vi "Curtin_FixJson.vi"(11 "String In":string) -> (3 "String out":string)   [LabVIEW 2022 SP3]
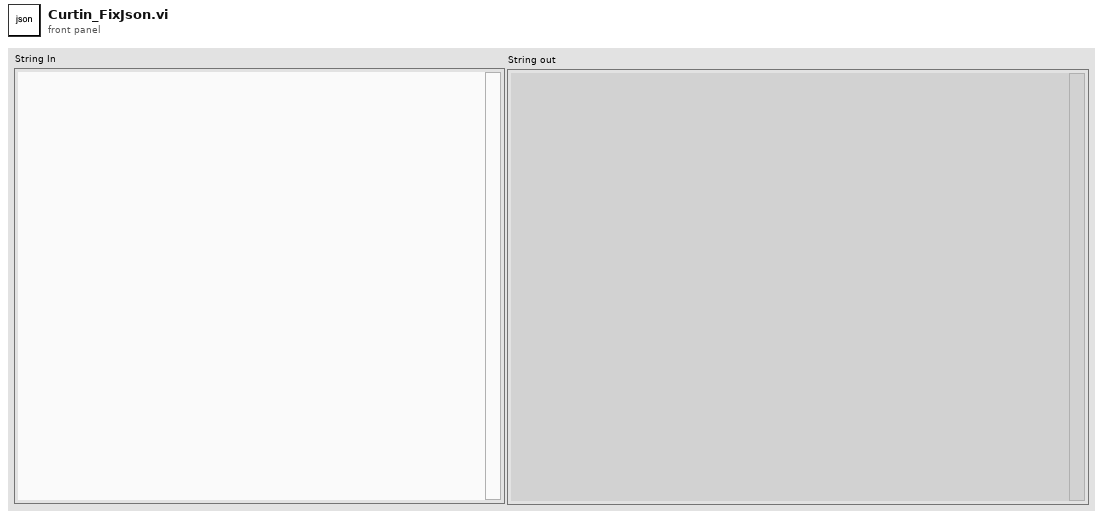
[diagram p1: front panel]
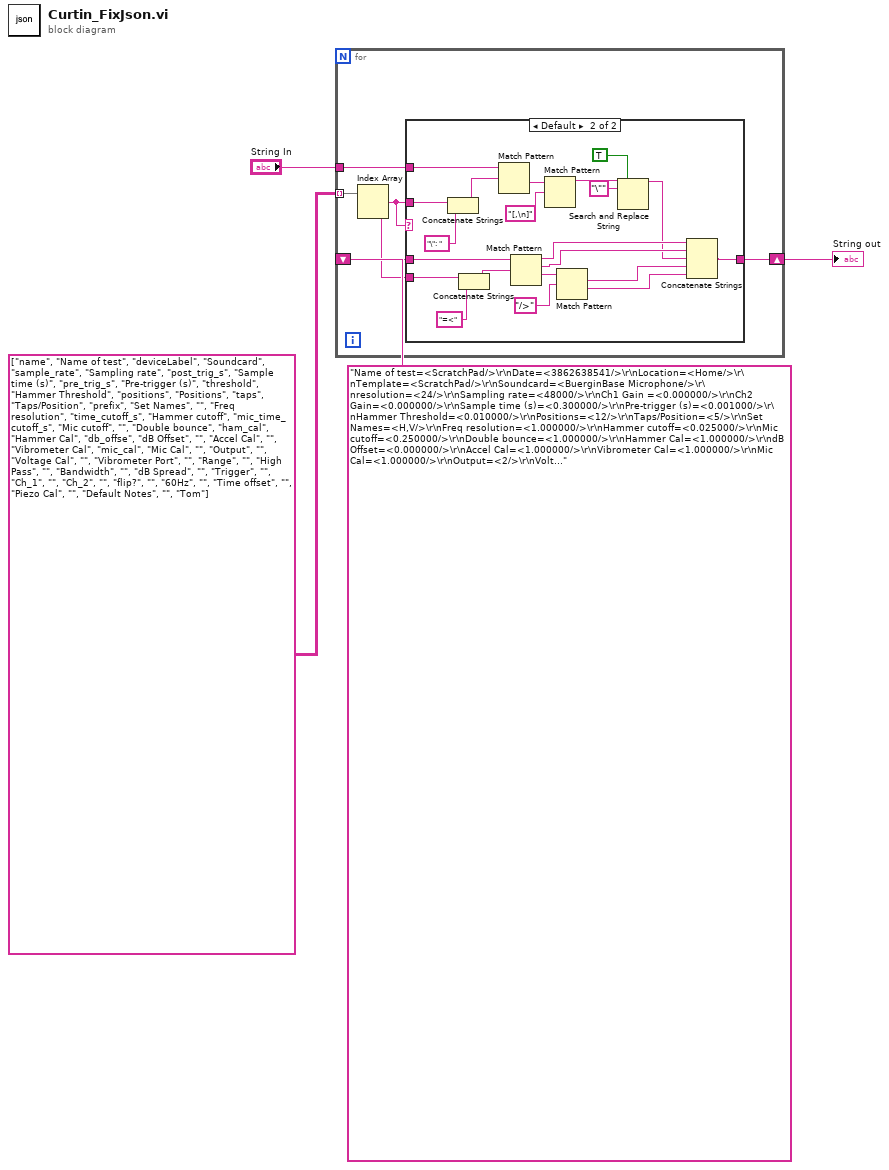
[diagram p0: block diagram]
diagram:
  n1 = for {
    tunnel: "String In" -> [w10]
    tunnel: string[][] [["name", "Name of test"], ["deviceLabel", "Soundcard"], ["sample_rate", "Sampling rate"], ["post_trig_s", "Sample time (s)"], ["pre_trig_s", "Pre-trigger (s)"], ["threshold", "Hammer Threshold"], ["positions", "Positions"], ["taps", "Taps/Position"], ["prefix", "Set Names"], ["", "Freq resolution"], ["time_cutoff_s", "Hammer cutoff"], ["mic_time_cutoff_s", "Mic cutoff"], ["", "Double bounce"], ["ham_cal", "Hammer Cal"], ["db_offse", "dB Offset"], ["", "Accel Cal"], ["", "Vibrometer Cal"], ["mic_cal", "Mic Cal"], ["", "Output"], ["", "Voltage Cal"], ["", "Vibrometer Port"], ["", "Range"], ["", "High Pass"], ["", "Bandwidth"], ["", "dB Spread"], ["", "Trigger"], ["", "Ch_1"], ["", "Ch_2"], ["", "flip?"], ["", "60Hz"], ["", "Time offset"], ["", "Piezo Cal"], ["", "Default Notes"], ["", "Tom"]] -> [w9] mode=indexing
    shift-right: [w6] -> w1
    shift-left: "Name of test=<ScratchPad/>\r\nDate=<3862638541/>\r\nLocation=<Home/>\r\nTemplate=<ScratchPad/>\r\nSoundcard=<BuerginBase Microphone/>\r\nresolution=<24/>\r\nSampling rate=<48000/>\r\nCh1 Gain =<0.000000/>\r\nCh2 Gain=<0.000000/>\r\nSample time (s)=<0.300000/>\r\nPre-trigger (s)=<0.001000/>\r\nHammer Threshold=<0.010000/>\r\nPositions=<12/>\r\nTaps/Position=<5/>\r\nSet Names=<H,V/>\r\nFreq resolution=<1.000000/>\r\nHammer cutoff=<0.025000/>\r\nMic cutoff=<0.250000/>\r\nDouble bounce=<1.000000/>\r\nHammer Cal=<1.000000/>\r\ndB Offset=<0.000000/>\r\nAccel Cal=<1.000000/>\r\nVibrometer Cal=<1.000000/>\r\nMic Cal=<1.000000/>\r\nOutput=<2/>\r\nVoltage Cal=<1.000000/>\r\nVibrometer Port=<ASRL27::INSTR/>\r\nRange=<50/>\r\nHigh Pass=<2/>\r\nBandwidth=<25/>\r\nX Range=<2.000000E+2\t1.000000E+4\t1.000000E+1\t1.000000E+2\t2.000000E+2\n0.000000E+0\t5.000000E-2\t2.500000E-2\t2.500000E-3\t0.000000E+0\n0.000000E+0\t3.000000E-1\t1.000000E-1\t1.000000E-2\t0.000000E+0\n2.000000E+2\t1.000000E+4\t1.000000E+1\t1.000000E+2\t1.000000E+3\n/>\r\nY Range=<-2.500000E+1\t0.000000E+0\t5.000000E+0\t1.000000E+0\t-2.500000E+1\n-1.000000E-1\t1.000000E+0\t2.500000E-1\t5.000000E-2\t0.000000E+0\n-1.000000E+0\t1.000000E+0\t5.000000E-1\t1.000000E-1\t-1.000000E+0\n-1.100000E+1\t2.900000E+1\t2.000000E+0\t5.000000E-1\t-1.000000E+1\n/>\r\ndB Spread=<40.000000/>\r\nTrigger=<0/>\r\nCh_1=<2/>\r\nCh_2=<1/>\r\nflip?=<false/>\r\n60Hz=<false/>\r\nTime offset=<0.000000/>\r\nPiezo Cal=<1.000000/>\r\nDefault Notes=<Instrument info: \n\n\n \nTemplate: HV 24  Obie 26\n\nMeasured at: \n\nMic: Behringer ECM 8000 at 20 cm\nSoundcard:  Mackie Onyx Producer 2.2 \n/>\r\nTom=<false/>\n" ("String Out") -> [w7]
    n2 = Index Array(array=w9) -> (element #1=w5:string, element #2=w8:string)  [unwired: 2 in]
    n3 = case shown="Default" w5 {
      tunnel: w10 -> [_ w32]
      tunnel: w5 -> [_ w30]
      tunnel: w8 -> [_ w27]
      tunnel: w7 -> [w11 w24]
      tunnel: [w11 w21] -> w6
      frame "" {
      }
      frame Default {
        n4 = Concatenate Strings(w30, "\": ") -> (w29:string)
        n5 = Concatenate Strings(w27, "=<") -> (w23:string)
        n6 = Match Pattern(string=w32, regular expression=w29) -> (after substring=w19:string)  [unwired: 1 in, 3 out]
        n7 = Match Pattern(string=w24, regular expression=w23) -> (before substring=w22:string, match substring=w17:string, after substring=w20:string)  [unwired: 1 in, 1 out]
        n8 = Match Pattern(string=w19, regular expression="[,\n]") -> (before substring=w15:string)  [unwired: 1 in, 3 out]
        n9 = Match Pattern(string=w20, regular expression="/>") -> (match substring=w16:string, after substring=w18:string)  [unwired: 1 in, 2 out]
        n10 = Search and Replace String(replace all?=TRUE ("replace all? (F)"), input string=w15, search string="\"") -> (result string=w14:string)  [unwired: 5 in, 3 out]
        n11 = Concatenate Strings(w22, w17, w14, w16, w18) -> (w21:string)
      }
    }
  }
  "String out" <- w1
